vi "read iKon Class.vi"(8 "error in (no error)":errorcluster, 11 "SPARC4_Channel in":refnum<class "ECHARPE_Channel.lvclass">) -> (0 "error out":errorcluster, 2 "iKon-L.lvclass":refnum<class "iKon-L.lvclass">, 3 "SPARC4_Channel out":refnum<class "ECHARPE_Channel.lvclass">)   [LabVIEW 2018, in "ECHARPE_Channel.lvclass"]
uses:
  ECHARPE_Channel.lvclass
  iKon-L/iKon-L.lvclass
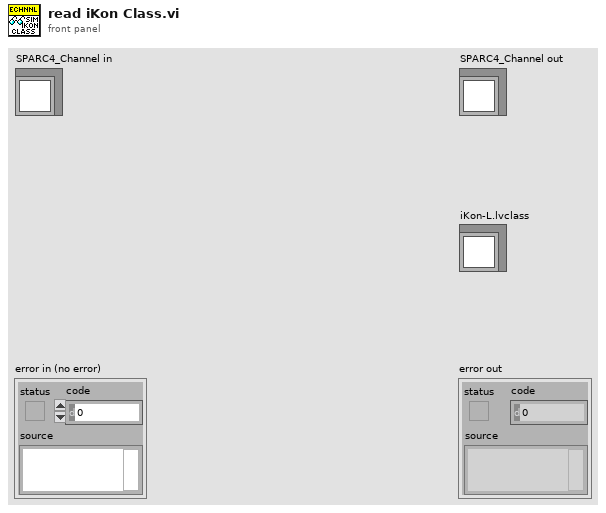
[diagram p1: front panel]
types:
  T1 = cluster{"State Machine.lvclass":refnum<class "State Machine.lvclass">, "RxTx.lvclass":refnum<class "RxTx.lvclass">, "Save_Header_RxTx.lvclass":refnum<class "RxTx.lvclass">, "Status SM.lvclass":refnum<class "State Machine.lvclass">, "Status RxTx.lvclass":refnum<class "RxTx.lvclass">, "servers array":refnum<class "Server.lvclass">[], "Events log file.lvclass":refnum<class "Log File.lvclass">, "Errors log file.lvclass":refnum<class "Log File.lvclass">, "Keywords log file.lvclass":refnum<class "Log File.lvclass">, "Sim_CCD.lvclass":refnum<class "Sim_CCD.lvclass">}
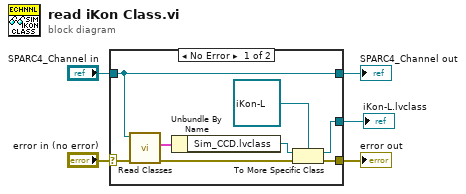
[diagram p0: block diagram]
diagram:
  n1 = case shown="No Error" "error in (no error)" {
    selector: "error in (no error)" -> [w13 w15]
    tunnel: [w7 w15] -> w4
    tunnel: [w12 w14] -> w2
    tunnel: "SPARC4_Channel in" -> [w12 w14]
    tunnel: [w9 _] -> w1
    frame No Error {
      n2 = call-dynamic "Read Classes.vi"("error in (no error)"=w13, "Channel in"=w12) -> ("error out"=w8:errorcluster, "Classes"=w11:T1)  [unwired: 7 in, 1 out]
      n3 = Unbundle By Name(w11) -> ("Sim_CCD.lvclass"=w10:refnum<class "Sim_CCD.lvclass">)
      n4 = To More Specific Class(target class=refnum<class "iKon-L.lvclass"> refnum ("iKon-L.lvclass"), reference=w10, error in=w8) -> (specific class reference=w9:refnum<class "iKon-L.lvclass">, error out=w7:errorcluster)
    }
    frame Error {
    }
  }
  "error out" <- w4
  "SPARC4_Channel out" <- w2
  "iKon-L.lvclass" <- w1
